vi "close.vi"(8 "error in (no error)":errorcluster caption="错误输入（无错误）", 11 "THM-V6数字型温湿度 输入":refnum<class "THM-V6数字型温湿度.lvclass">) -> (0 "error out":errorcluster caption="错误输出", 3 "THM-V6数字型温湿度 输出":refnum<class "THM-V6数字型温湿度.lvclass">)   [LabVIEW 2016, in "THM-V6数字型温湿度.lvlib" / "THM-V6数字型温湿度.lvclass"]
uses:
  <vilib>/Plasmionique/MB Master/MB_Master/MB_Master.lvclass
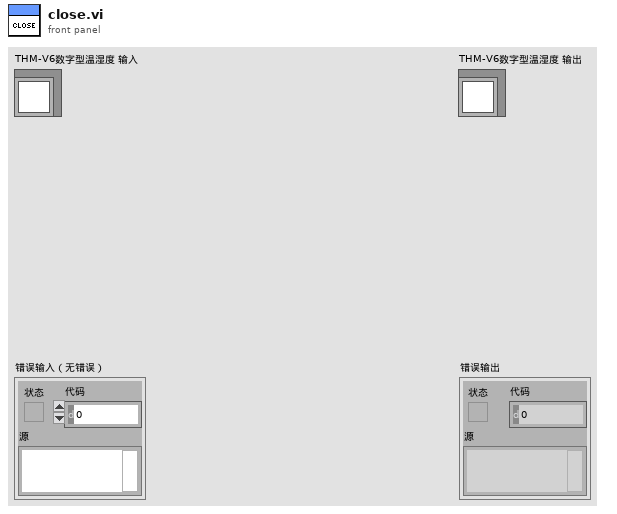
[diagram p1: front panel]
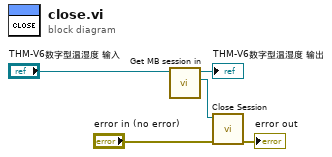
[diagram p0: block diagram]
diagram:
  n1 = call "Get MB session in.vi"("THM-V6数字型温湿度 in"="THM-V6数字型温湿度 输入") -> ("MB Serial Master:MB_Master"=w4:refnum<class "MB_Master.lvclass">, "THM-V6数字型温湿度 out"=→"THM-V6数字型温湿度 输出":refnum<class "THM-V6数字型温湿度.lvclass">)  [unwired: 9 in]
  n2 = call-dynamic "Close Session.vi"("error in (no error)"="error in (no error)", "MB session in"=w4) -> ("error out"=→"error out":errorcluster)  [unwired: 9 in]
